vi "Main.vi"(11 "Module Admin":refnum<class "Delacor_lib_QMH_Module Admin.lvclass">) -> ()   [LabVIEW 2024, in "GUI.lvlib"]
doc: "This template is based off of the Queued Message Handler design pattern and the Queued Message Handler project template that ships with LabVIEW.\n\nThe main difference is that the queue is private to this module and communication between modules is performed via Broadcast and Request events.\n\nRequest events are wrapped in public API methods and are handled in the Event Handling Loop (EHL) of this VI. Any module can register for Broadcast events sent by this module. The EHL generates messages based on user interface actions.\n\nThe Message Handling Loop (MHL) processes messages generated by the EHL, or by other messages. The messages are string values, so new messages can be added easily to the Message Cases case structure in the MHL. Each message cluster can also provide an optional value for Message Data, which is a variant that can be converted to whatever message-specific data is required.\n_____\nBased on DQMH Project Template 7.0.1.1316."
uses:
  GUI.lvlib
  <vilib>/Delacor/Delacor QMH/Libraries/Module Admin_class/Delacor_lib_QMH_Module Admin.lvclass
  Module Data--cluster.ctl
  <vilib>/Delacor/Delacor QMH/Libraries/Message Queue_class/Delacor_lib_QMH_Message Queue.lvclass/Delacor_lib_QMH_Message Queue.ctl
  Stop Argument--cluster.ctl
  <vilib>/Delacor/Delacor QMH/Libraries/Module Admin_class/Delacor_lib_QMH_Module Admin.lvclass/Delacor_lib_QMH_Module Admin.ctl
  <vilib>/Utility/miscctls.llb/LVPointTypeDef.ctl
  <vilib>/Delacor/Delacor QMH/Libraries/Message Queue_class/Delacor_lib_QMH_Enqueue Message (Single).vi
  <vilib>/Delacor/Delacor QMH/Libraries/Module Admin_class/Delacor_lib_QMH_Get External Launch.vi
  <vilib>/Delacor/Delacor QMH/Libraries/Message Queue_class/Delacor_lib_QMH_Message Queue.lvclass
  <vilib>/addons/_JKI.lib/REST Client/classes/REST Client/REST Client.lvclass
  <vilib>/NI/Advanced HTTP Client/Header--Combo Box.ctl
  <vilib>/NI/Advanced HTTP Client/Session.lvclass
  <vilib>/addons/_JKI.lib/REST Client/classes/REST Client/HTTP Header.ctl
panel:
  in  "Current Status":bool
  out "error out":errorcluster
  out "Status":string
  in  "Simulate MHL Error":bool
  in  "Simulate EHL Error":bool
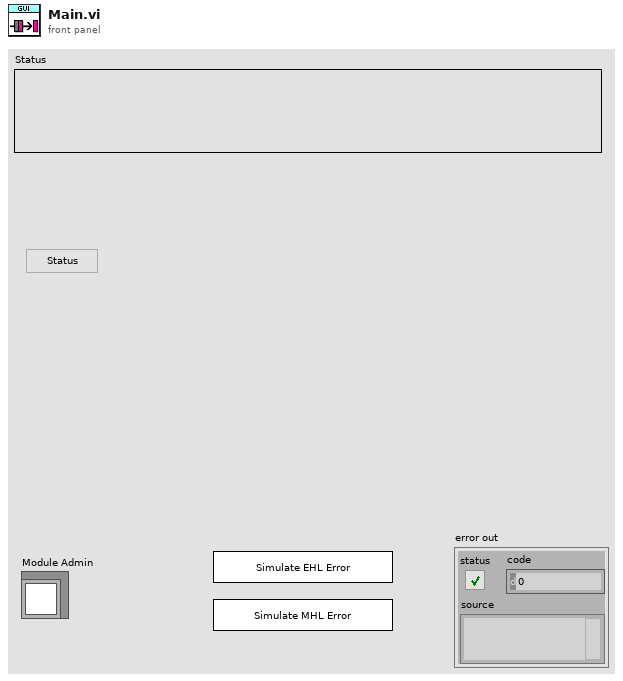
[diagram p1: front panel]
types:
  T1 = typedef "GUI.lvlib/Request Events--cluster.ctl" = cluster{"Stop Module":refnum<user-event>, "Show Panel":refnum<user-event>, "Hide Panel":refnum<user-event>, "Get Module Execution Status":refnum<user-event>, "Show Diagram":refnum<user-event>}
  T2 = typedef "GUI.lvlib/Module Data--cluster.ctl" = cluster{"Status":string, "Token":string, "Root Path":string, "REST Client":refnum<class "REST Client.lvclass">}
  T3 = enum32{"invalid lock state", "Not Locked", "Locked (No Password)", "Password-protected"}
  T4 = typedef "GUI.lvlib/Stop Argument--cluster.ctl" = cluster{"Origin":string, "Exit via Stop Module Req?":bool, "Wait for Module to stop?":bool}
  T5 = typedef "LVPointTypeDef.ctl" = cluster{"Horizontal":i16, "Vertical":i16}
  T6 = enum32{"Invalid", "Standard", "Closed", "Hidden", "Minimized", "Maximized"}
  T7 = typedef "lib_NI_Advanced HTTP Client.lvlib/Session.lvclass/Header--Combo Box.ctl" = string
  T8 = typedef "REST Client.lvlib/REST Client.lvclass/HTTP Header.ctl" = cluster{"header":T7, "value":string}
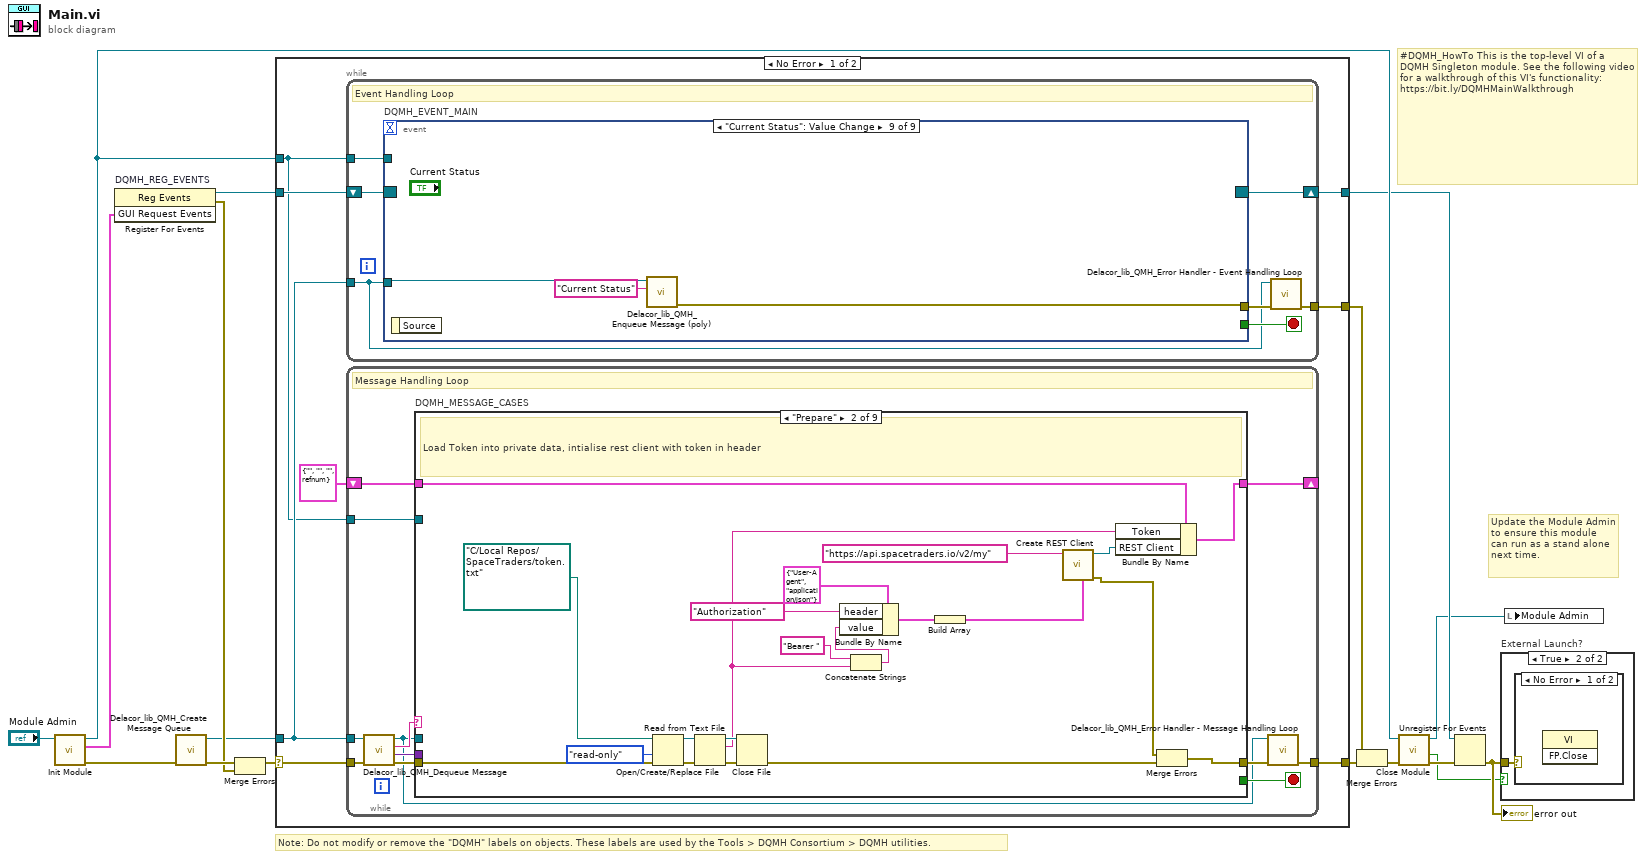
[diagram p0: block diagram]
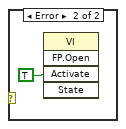
[diagram p3: hidden frame]
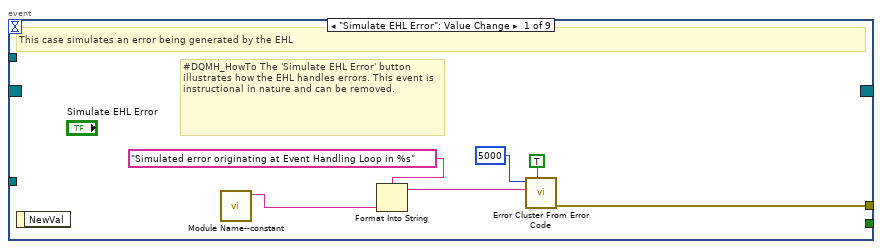
[diagram p4: hidden frame]
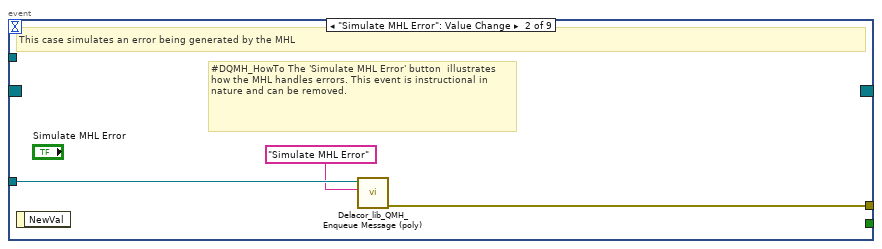
[diagram p5: hidden frame]
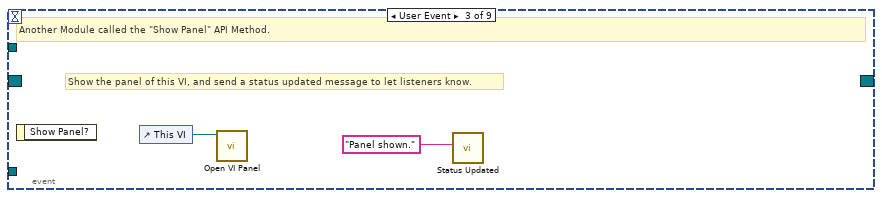
[diagram p6: hidden frame]
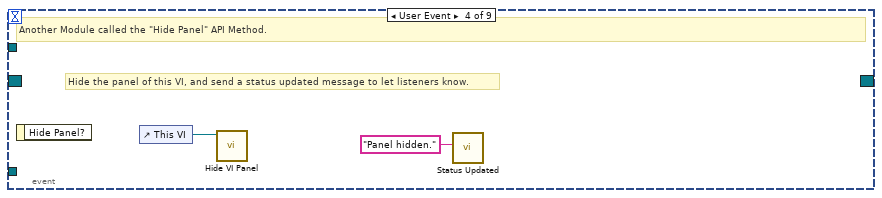
[diagram p7: hidden frame]
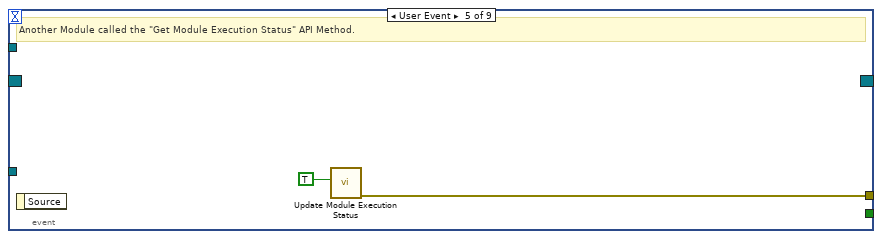
[diagram p8: hidden frame]
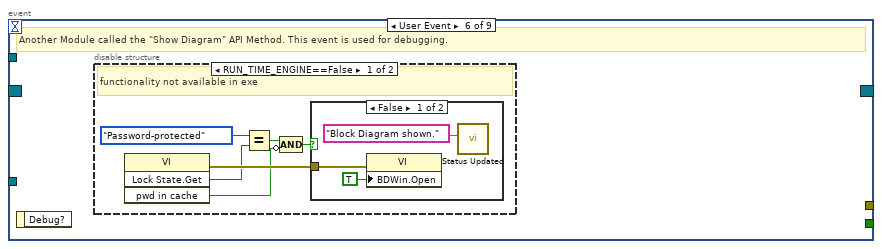
[diagram p9: hidden frame]
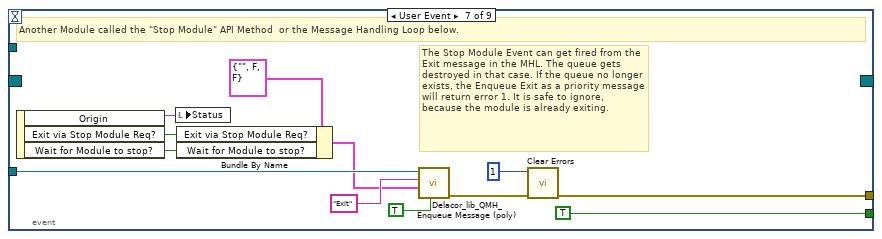
[diagram p12: hidden frame]
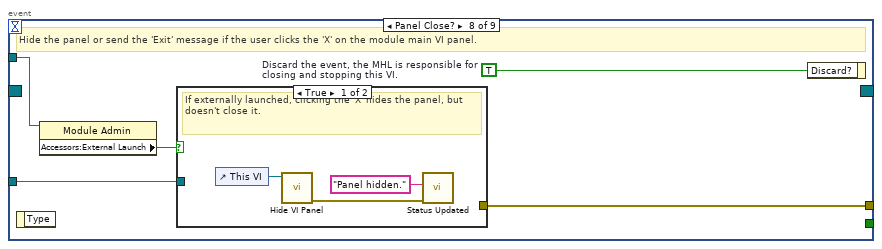
[diagram p13: hidden frame]
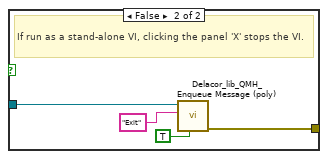
[diagram p14: hidden frame]
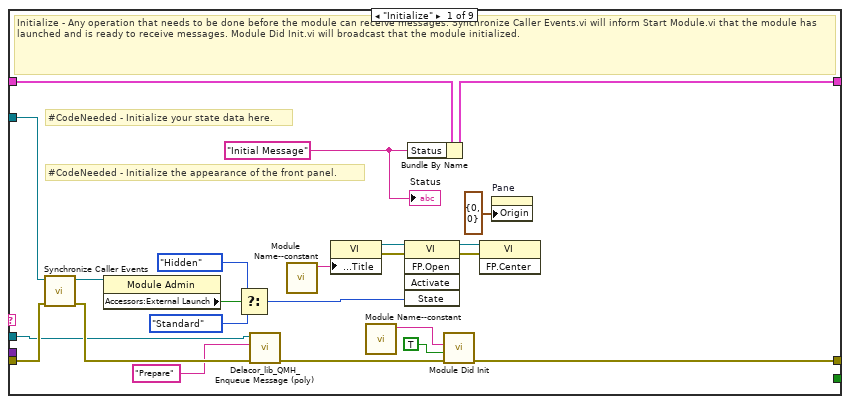
[diagram p15: hidden frame]
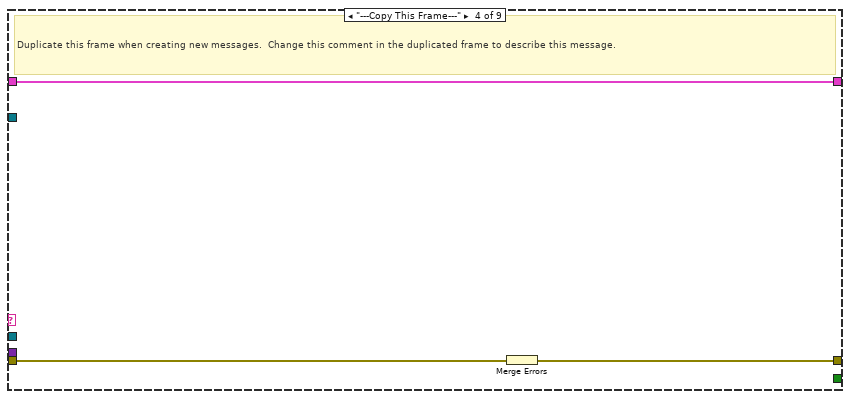
[diagram p17: hidden frame]
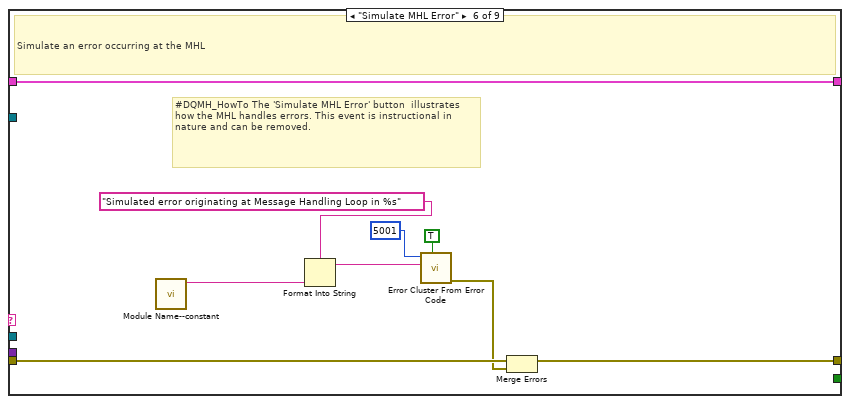
[diagram p19: hidden frame]
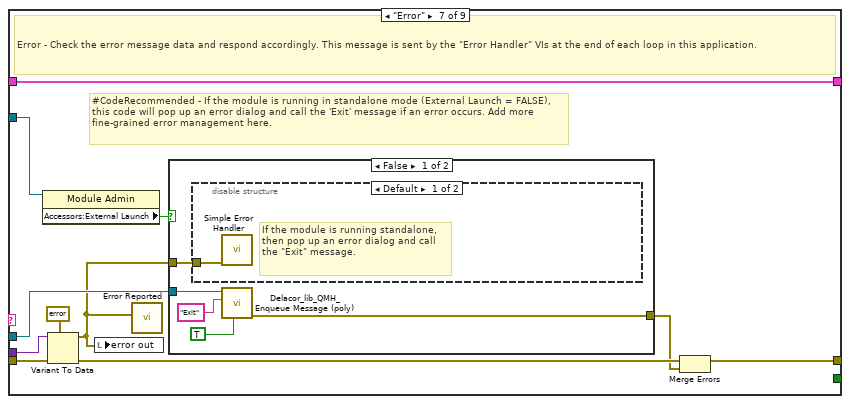
[diagram p20: hidden frame]
diagram:
  # "#DQMH_HowTo This is the top-level VI of a DQMH Singleton module. See the following video for a walkthrough of this VI's functionality: https://bit.ly/DQMHMainWalkthrough"
  # "Note: Do not modify or remove the \"DQMH\" labels on objects. These labels are used by the Tools > DQMH Consortium > DQMH utilities."
  # "Update the Module Admin to ensure this module can run as a stand alone next time."
  n1 = call "Init Module.vi"("Singleton Module Admin in"="Module Admin") -> ("error out"=w16:errorcluster, "GUI Request Events"=w5:T1, "Singleton Module Admin out"=w8:refnum<class "Delacor_lib_QMH_Module Admin.lvclass">)  [unwired: 8 in]
  n2 = register-events "DQMH_REG_EVENTS"(w5) -> (reference out=w6:refnum<event-registration>, error out=w9:errorcluster)  [unwired: 2 in]
  n3 = call <vilib>:"Delacor_lib_QMH_Create Message Queue.vi"("error in"=w16) -> ("error out"=w11:errorcluster, "Message Queue"=w4:refnum<class "Delacor_lib_QMH_Message Queue.lvclass">)  [unwired: 9 in]
  n4 = Merge Errors(w11, w9) -> (w10:errorcluster)
  n5 = case shown="No Error" w10 {
    selector: w10 -> [w23 w206]
    tunnel: [w25 w205] -> w17
    tunnel: [w22 w204] -> w7
    tunnel: w6 -> [w20 w204]
    tunnel: w4 -> [w19 w199]
    tunnel: [w24 _] -> w14
    tunnel: w8 -> [w18 w200]
    frame No Error {
      n6 = while {
        tunnel: w19 -> [w26]
        shift-right: [w29] -> w22
        shift-left: w20 -> [w30]
        tunnel: [w31] -> w24
        tunnel: w18 -> [w27]
        stop <- w28 stop-if-true
        # "Event Handling Loop"
        n7 = event "DQMH_EVENT_MAIN" shown="[8] \"Current Status\": Value Change" {
          selector: w30 -> [_ _ _ _ _ _ _ _ _]
          dyn-events: [_ _ _ _ _ _ _ _ _] -> w29
          timeout: _ -> [_ _ _ _ _ _ _ _ _]
          tunnel: [_ _ _ _ _ _ TRUE ("Discard?") _ _] -> w28
          tunnel: w26 -> [_ w40 _ _ _ _ w64 w71 w83]
          tunnel: [w38 w41 _ _ w47 _ w67 w73 w82] -> w32
          tunnel: w27 -> [_ _ _ _ _ _ _ w70 _]
          event "Simulate EHL Error": Value Change {
            # "#DQMH_HowTo The 'Simulate EHL Error' button  illustrates how the EHL handles errors. This event is instructional in nature and can be removed."
            # "This case simulates an error being generated by the EHL"
            n8 = event-data() -> ()  [unwired: 1 in, 1 out]
            n9 = call "Module Name--constant.vi"() -> ("Module Name"=w35:string)  [unwired: 11 in]
            n10 = Format Into String(format string="Simulated error originating at Event Handling Loop in %s", w35) -> (resulting string=w36:string)  [unwired: 2 in, 1 out]
            n11 = call <vilib>:"Error Cluster From Error Code.vi"("show call chain? (False)"=TRUE, "error message (\"\")"=w36, "error code (0)"=5000) -> ("error out"=w38:errorcluster)  [unwired: 6 in]
          }
          event "Simulate MHL Error": Value Change {
            # "#DQMH_HowTo The 'Simulate MHL Error' button  illustrates how the MHL handles errors. This event is instructional in nature and can be removed."
            # "This case simulates an error being generated by the MHL"
            n12 = event-data() -> ()  [unwired: 1 in, 1 out]
            n13 = call-poly <vilib>:"Delacor_lib_QMH_Enqueue Message (poly).vi"("Message"="Simulate MHL Error", "Message Queue in"=w40) -> ("error out"=w41:errorcluster)  [unwired: 8 in, 1 out]
          }
          event User Event {
            # "Show the panel of this VI, and send a status updated message to let listeners know."
            # "Another Module called the \"Show Panel\" API Method."
            n14 = event-data() -> ()  [unwired: 1 in, 1 out]
            n15 = control-ref of="This VI"() -> (w43:refnum<vi>)
            n16 = call "Open VI Panel.vi"("VI"=w43) -> ()  [unwired: 10 in, 1 out]
            n17 = call "Status Updated.vi"("Status"="Panel shown." ("format string")) -> ()  [unwired: 10 in, 1 out]
          }
          event User Event {
            # "Hide the panel of this VI, and send a status updated message to let listeners know."
            # "Another Module called the \"Hide Panel\" API Method."
            n18 = event-data() -> ()  [unwired: 1 in, 1 out]
            n19 = control-ref of="This VI"() -> (w45:refnum<vi>)
            n20 = call "Hide VI Panel.vi"("VI"=w45) -> ()  [unwired: 10 in, 1 out]
            n21 = call "Status Updated.vi"("Status"="Panel hidden." ("format string")) -> ()  [unwired: 10 in, 1 out]
          }
          event User Event {
            # "Another Module called the \"Get Module Execution Status\" API Method."
            n22 = event-data() -> ()  [unwired: 1 in, 1 out]
            n23 = call "Update Module Execution Status.vi"("Running?"=TRUE) -> ("error out"=w47:errorcluster)  [unwired: 10 in]
          }
          event User Event {
            # "Another Module called the \"Show Diagram\" API Method. This event is used for debugging."
            n24 = event-data() -> ()  [unwired: 1 in, 1 out]
            n25 = disable-structure shown="RUN_TIME_ENGINE==False" {
              frame condition #0 (active) {
                # "functionality not available in exe"
                n26 = invoke on="Invoke Node" class="VI" method="Lock State.Get"() -> (error out=w53:errorcluster, "Get Lock State"=w52:T3, "pwd in cache"=w49:bool)  [unwired: 4 in, 1 out]
                n27 = Equal?(x=T3."Password-protected", y=w52) -> (x = y?=w50:bool)
                n28 = Compound Arithmetic op=AND(w50, invert w49) -> (w48:bool)
                n29 = case shown="False" w48 {
                  tunnel: w53 -> [w56 _]
                  frame False {
                    n30 = property on="Property Node" class="VI"(error in=w56, "BDWin.Open"=TRUE ("Block Diagram Window:Open")) -> ()  [unwired: 1 in, 2 out]
                    n31 = call "Status Updated.vi"("Status"="Block Diagram shown." ("format string")) -> ()  [unwired: 10 in, 1 out]
                  }
                  frame True {
                    # "Password-protected VI, and the password is not in the cache. Do not show the diagram."
                  }
                }
              }
              frame condition #1 {
              }
            }
          }
          event User Event {
            # "The Stop Module Event can get fired from the Exit message in the MHL. The queue gets destroyed in that case. If the queue no longer exists, the Enqueue Exit as a priority message will return error 1. It is safe to ignore, because the module is already exiting."
            # "Another Module called the \"Stop Module\" API Method  or the Message Handling Loop below."
            n32 = event-data() -> ("Origin"=w63:string, "Exit via Stop Module Req?"=w59:bool, "Wait for Module to stop?"=w58:bool)  [unwired: 1 in]
            n33 = local write "Status"(w63) -> ()
            n34 = Bundle By Name(cluster=T4 {"Origin"="", "Exit via Stop Module Req?"=FALSE, "Wait for Module to stop?"=FALSE} ("Stop Argument"), "Exit via Stop Module Req?"=w59, "Wait for Module to stop?"=w58) -> (w57:T4)
            n35 = call-poly <vilib>:"Delacor_lib_QMH_Enqueue Message (poly).vi"("Priority Message? (F)"=TRUE, "Message Data"=w57, "Message"="Exit", "Message Queue in"=w64) -> ("error out"=w68:errorcluster)  [unwired: 6 in, 1 out]
            n36 = call <vilib>:"Clear Errors.vi"("error in (no error)"=w68, "specific error code to clear (0: all)"=1) -> ("error out"=w67:errorcluster)  [unwired: 4 in, 1 out]
          }
          event Panel Close? {
            w72 = TRUE  # Discard the event, the MHL is responsible for closing and stopping this VI.
            # "Hide the panel or send the 'Exit' message if the user clicks the 'X' on the module main VI panel."
            n37 = event-data() -> ()  [unwired: 1 in, 1 out]
            n38 = property on="Property Node" class="Module Admin"(reference=w70) -> ("Accessors:External Launch"=w69:bool)  [unwired: 1 in, 2 out]
            n39 = case shown="True" w69 {
              tunnel: w71 -> [_ w79]
              tunnel: [_ w80] -> w73
              frame True {
                # "If externally launched, clicking the 'X' hides the panel, but doesn't close it."
                n40 = control-ref of="This VI"() -> (w76:refnum<vi>)
                n41 = call "Hide VI Panel.vi"("VI"=w76) -> ("error out"=w74:errorcluster)  [unwired: 10 in]
                n42 = call "Status Updated.vi"("error in"=w74, "Status"="Panel hidden." ("format string")) -> ()  [unwired: 9 in, 1 out]
              }
              frame False {
                # "If run as a stand-alone VI, clicking the panel 'X' stops the VI."
                n43 = call-poly <vilib>:"Delacor_lib_QMH_Enqueue Message (poly).vi"("Priority Message? (F)"=TRUE, "Message"="Exit", "Message Queue in"=w79) -> ("error out"=w80:errorcluster)  [unwired: 7 in, 1 out]
              }
            }
            n44 = event-data ("Event Filter Node")("Discard?"=w72) -> ()  [unwired: 1 in, 1 out]
          }
          event "Current Status": Value Change {
            n45 = event-data() -> ()  [unwired: 1 in, 1 out]
            n46 = call-poly <vilib>:"Delacor_lib_QMH_Enqueue Message (poly).vi"("Message"="Current Status", "Message Queue in"=w83) -> ("error out"=w82:errorcluster)  [unwired: 8 in, 1 out]
          }
        }
        n47 = call-dynamic "Delacor_lib_QMH_Error Handler - Event Handling Loop.vi"("error in"=w32, "Message Queue in"=w26) -> ("dup error in"=w31:errorcluster)  [unwired: 8 in, 1 out]
      }
      n48 = while {
        tunnel: w19 -> [w84]
        shift-right: [w92] -> _
        shift-left: T2 {"Status"="", "Token"="", "Root Path"="", "REST Client"=refnum} ("Data Cluster") -> [w93]
        tunnel: w23 -> [w95]
        tunnel: [w87] -> w25
        tunnel: w18 -> [w88]
        stop <- w91 stop-if-true
        # "Message Handling Loop"
        n49 = call-dynamic "Delacor_lib_QMH_Dequeue Message.vi"("error in"=w95, "Message Queue in"=w84) -> ("error out"=w94:errorcluster, "Message Data"=w89:variant, "Message"=w90:string, "Message Queue out"=w85:refnum<class "Delacor_lib_QMH_Message Queue.lvclass">)  [unwired: 6 in]
        n50 = case "DQMH_MESSAGE_CASES" shown="\"Prepare\"" w90 {
          selector: w90 -> [_ _ _ _ _ _ _ _ w194]
          tunnel: w85 -> [w97 _ _ _ _ _ w159 w182 _]
          tunnel: w94 -> [w116 w131 w141 w144 w146 w155 w166 w188 w197]
          tunnel: [w114 w127 w141 w143 w146 w154 w162 w183 w198] -> w86
          tunnel: w93 -> [w105 w134 w140 w142 w145 w152 w161 w174 w195]
          tunnel: [w104 w133 w140 w142 w145 w152 w161 w174 w195] -> w92
          tunnel: [_ _ _ _ _ _ _ w181 _] -> w91
          tunnel: w89 -> [_ _ _ _ _ _ w160 w180 _]
          tunnel: w88 -> [w106 _ _ _ _ _ w158 w175 _]
          frame "Initialize" {
            w100 = "Initial Message" ("Initial Message")
            # "#CodeNeeded - Initialize the appearance of the front panel."
            # "#CodeNeeded - Initialize your state data here."
            # "Initialize - Any operation that needs to be done before the module can receive messages. Synchronize Caller Events.vi will inform Start Module.vi that the module has launched and is ready to receive messages. Module Did Init.vi will broadcast that the module initialized."
            n51 = call "Synchronize Caller Events.vi"("error in"=w116, "Singleton Module Admin in"=w106) -> ("error out"=w115:errorcluster, "Singleton Module Admin out"=w101:refnum<class "Delacor_lib_QMH_Module Admin.lvclass">)  [unwired: 8 in]
            n52 = property on="Property Node" class="Module Admin"(reference=w101) -> ("Accessors:External Launch"=w110:bool)  [unwired: 1 in, 2 out]
            n53 = Select(t=T6."Hidden" ("State"), s=w110, f=T6."Standard" ("State")) -> (s? t:f=w107:T6)
            n54 = call-poly <vilib>:"Delacor_lib_QMH_Enqueue Message (poly).vi"("error in"=w115, "Message"="Prepare", "Message Queue in"=w97) -> ("error out"=w98:errorcluster)  [unwired: 7 in, 1 out]
            n55 = call "Module Name--constant.vi"() -> ("Module Name"=w113:string)  [unwired: 11 in]
            n56 = property on="Property Node" class="VI"("Front Panel.Title"=w113) -> (reference out=w112:refnum<vi>, error out=w118:errorcluster)  [unwired: 2 in]
            n57 = call "Module Name--constant.vi"() -> ("Module Name"=w102:string)  [unwired: 11 in]
            n58 = invoke on="Invoke Node" class="VI" method="FP.Open"(reference=w112, error in=w118, "State"=w107) -> (reference out=w111:refnum<vi>, error out=w117:errorcluster)  [unwired: 2 in, 3 out]
            n59 = Bundle By Name(cluster=w105, "Status"=w100) -> (w104:T2)
            n60 = call "Module Did Init.vi"("error in"=w98, "Initialized?"=TRUE, "Origin"=w102) -> ("error out"=w114:errorcluster)  [unwired: 8 in]
            n61 = invoke on="Invoke Node" class="VI" method="FP.Center"(reference=w111, error in=w117) -> ()  [unwired: 1 in, 3 out]
            n62 = property on="Pane" class="Pane"("Origin"=T5 {"Horizontal"=0, "Vertical"=0}) -> ()  [unwired: 2 in, 2 out]
            "Status" <- w100
          }
          frame "Prepare" {
            # "Load Token into private data, intialise rest client with token in header"
            n63 = Open/Create/Replace File(file path (use dialog)=path "C:/Local Repos/SpaceTraders/token.txt", error in=w131, access (0:read/write)=enum16{"read/write", "read-only", "write-only"}."read-only") -> (refnum out=w139:refnum<file>, error out=w138:errorcluster)  [unwired: 3 in, 1 out]
            n64 = Read from Text File(file (use dialog)=w139, error in=w138) -> (refnum out=w137:refnum<file>, text=w119:string, error out=w136:errorcluster)  [unwired: 2 in, 1 out]
            n65 = Close File(refnum=w137, error in=w136) -> (error out=w132:errorcluster)  [unwired: 1 out]
            n66 = Concatenate Strings("Bearer ", w119) -> (w121:string)
            n67 = Bundle By Name(cluster=T8 {"header"="User-Agent", "value"="application/json"} ("Header"), "header"=T7 "Authorization", "value"=w121) -> (w123:T8)
            n68 = Build Array(w123) -> (w122:T8[])
            n69 = call <vilib>:"Create REST Client.vi"("Default Headers ([JSON])"=w122, "Base URL"="https://api.spacetraders.io/v2/my" ("Root Path")) -> ("error out"=w126:errorcluster, "REST Client out"=w128:refnum<class "REST Client.lvclass">)  [unwired: 8 in]
            n70 = Bundle By Name(cluster=w134, "Token"=w119, "REST Client"=w128) -> (w133:T2)
            n71 = Merge Errors(w126, w132) -> (w127:errorcluster)
          }
          frame "---Module Specific---" {
            # "Separator -- The following cases handle messages specific to this Module."
          }
          frame "---Copy This Frame---" {
            # "Duplicate this frame when creating new messages.  Change this comment in the duplicated frame to describe this message."
            n72 = Merge Errors(w144) -> (w143:errorcluster)
          }
          frame "---Exit and Error Handling---" {
            # "Separator - The following cases handle errors and exit messages."
          }
          frame "Simulate MHL Error" {
            # "#DQMH_HowTo The 'Simulate MHL Error' button  illustrates how the MHL handles errors. This event is instructional in nature and can be removed."
            # "Simulate an error occurring at the MHL"
            n73 = call "Module Name--constant.vi"() -> ("Module Name"=w148:string)  [unwired: 11 in]
            n74 = Format Into String(format string="Simulated error originating at Message Handling Loop in %s", w148) -> (resulting string=w149:string)  [unwired: 2 in, 1 out]
            n75 = call <vilib>:"Error Cluster From Error Code.vi"("show call chain? (False)"=TRUE, "error message (\"\")"=w149, "error code (0)"=5001) -> ("error out"=w153:errorcluster)  [unwired: 6 in]
            n76 = Merge Errors(w155, w153) -> (w154:errorcluster)
          }
          frame "Error" {
            # "#CodeRecommended - If the module is running in standalone mode (External Launch = FALSE), this code will pop up an error dialog and call the 'Exit' message if an error occurs. Add more fine-grained error management here."
            # "Error - Check the error message data and respond accordingly. This message is sent by the \"Error Handler\" VIs at the end of each loop in this application."
            n77 = property on="Property Node" class="Module Admin"(reference=w158) -> ("Accessors:External Launch"=w157:bool)  [unwired: 1 in, 2 out]
            n78 = Variant To Data(error in=w166, type=errorcluster {"status"=FALSE, "code"=0, "source"=""} ("error constant"), Variant=w160) -> (data=w156:errorcluster, error out=w164:errorcluster)
            n79 = local write "error out"(w156) -> ()
            n80 = call "Error Reported.vi"("Error"=w156) -> ()  [unwired: 10 in, 1 out]
            n81 = case shown="False" w157 {
              tunnel: [w171 _] -> w163
              tunnel: w159 -> [w169 _]
              tunnel: w156 -> [w170 _]
              frame False {
                n82 = disable-structure shown="Default" {
                  disable-tunnel: w170 -> [w172 _]
                  frame condition #0 (active) {
                    # "If the module is running standalone, then pop up an error dialog and call the \"Exit\" message."
                    n83 = call <vilib>:"Simple Error Handler.vi"("error in (no error)"=w172) -> ()  [unwired: 4 in, 5 out]
                  }
                  frame condition #1 {
                    # "To prevent the Simple Error Handler VI from being loaded (e.g. when deploying to a Real-Time target), add the Conditional Disable Symbol \"DQMH_Disable_SEH\" to your project and set it to TRUE."
                  }
                }
                n84 = call-poly <vilib>:"Delacor_lib_QMH_Enqueue Message (poly).vi"("Priority Message? (F)"=TRUE, "Message"="Exit", "Message Queue in"=w169) -> ("error out"=w171:errorcluster)  [unwired: 7 in, 1 out]
              }
              frame True {
                # "If the module was launched externally, calling the Error Reported broadcast VI is the only action performed by the \"Error\" message. The module's caller can then process the error appropriately."
              }
            }
            n85 = Merge Errors(w164, w163) -> (w162:errorcluster)
          }
          frame "Exit" {
            w179 = 91  # 91: not all Exit messages will have an argument
            w181 = TRUE  # Stop the VI
            # "Release the message queue reference"
            # "#CodeNeeded - Add any required cleanup code here."
            # "Exit - Exit the application."
            n86 = Variant To Data(error in=w188, type=T4 {"Origin"="", "Exit via Stop Module Req?"=FALSE, "Wait for Module to stop?"=FALSE} ("Stop Argument"), Variant=w180) -> (data=w177:T4, error out=w185:errorcluster)
            n87 = call <vilib>:"Clear Errors.vi"("error in (no error)"=w185, "specific error code to clear (0: all)"=w179) -> ("error out"=w187:errorcluster)  [unwired: 4 in, 1 out]
            n88 = control-ref of="This VI"() -> (w176:refnum<vi>)
            n89 = call-dynamic "Delacor_lib_QMH_Release Message Queue.vi"("error in"=w187, "Message Queue"=w182) -> ("error out"=w186:errorcluster)  [unwired: 9 in]
            n90 = call "Handle Exit.vi"("Stop Argument"=w177, "Admin in"=w175, "VI reference"=w176) -> ("error out"=w184:errorcluster)  [unwired: 7 in, 1 out]
            n91 = Merge Errors(w186, w184) -> (w183:errorcluster)
            n92 = Unbundle By Name(w174) -> ("REST Client"=w173:refnum<class "REST Client.lvclass">)
            n93 = call "Error Reported.vi"("Error"=w183) -> ()  [unwired: 10 in, 1 out]
            n94 = call-dynamic "Destroy REST Client.vi"("REST Client in"=w173) -> ()  [unwired: 10 in, 1 out]
          }
          frame Default {
            # "'Default' case only runs if there is a message that isn't defined in any of the other cases.  Output a programming error."
            n95 = call "Module Name--constant.vi"() -> ("Module Name"=w193:string)  [unwired: 11 in]
            n96 = Format Into String(format string="The invalid message string \"%s\" was received in the Message Handling Loop for module \"%s\".", w194, w193) -> (resulting string=w189:string)  [unwired: 2 in, 1 out]
            n97 = call <vilib>:"Error Cluster From Error Code.vi"("show call chain? (False)"=TRUE, "error message (\"\")"=w189, "error code (0)"=1) -> ("error out"=w196:errorcluster)  [unwired: 6 in]
            n98 = Merge Errors(w197, w196) -> (w198:errorcluster)
          }
        }
        n99 = call-dynamic "Delacor_lib_QMH_Error Handler - Message Handling Loop.vi"("error in"=w86, "Message Queue in"=w85) -> ("dup error in"=w87:errorcluster)  [unwired: 8 in, 1 out]
      }
    }
    frame Error {
      # "Synchronize Caller Events.vi will inform Start Module.vi that the module has launched and will let the code calling Start Module.vi register for broadcasts and would permit the caller receive the broadcast that an error occurred at launch time."
      n100 = call-dynamic "Delacor_lib_QMH_Release Message Queue.vi"("error in"=w206, "Message Queue"=w199) -> ("error out"=w205:errorcluster)  [unwired: 9 in]
      n101 = call "Synchronize Caller Events.vi"("Singleton Module Admin in"=w200) -> ("error out"=w207:errorcluster)  [unwired: 9 in, 1 out]
      n102 = call "Module Name--constant.vi"() -> ("Module Name"=w203:string)  [unwired: 11 in]
      n103 = Format Into String(format string="An error occurred during initialization. %s is no longer running.", w203) -> (resulting string=w201:string)  [unwired: 2 in, 1 out]
      n104 = Merge Errors(w205, w207) -> (w208:errorcluster)
      n105 = call "Error Reported.vi"("Additional Information"=w201, "Error"=w208) -> ()  [unwired: 9 in, 1 out]
    }
  }
  n106 = Merge Errors(w14, w17) -> (w13:errorcluster)
  n107 = call "Close Module.vi"("error in"=w13, "Module Admin in"=w8) -> ("error out"=w15:errorcluster, "External Launch"=w1:bool, "Module Admin out"=w2:refnum<class "Delacor_lib_QMH_Module Admin.lvclass">)  [unwired: 7 in]
  n108 = Unregister For Events(event registration refnum=w7, error in=w15) -> (error out=w12:errorcluster)
  "error out" <- w12
  n109 = case "External Launch?" shown="True" w1 {
    tunnel: w12 -> [_ w209]
    frame False {
    }
    frame True {
      n110 = case shown="No Error" w209 {
        frame No Error {
          n111 = invoke on="Invoke Node" class="VI" method="FP.Close"() -> ()  [unwired: 3 in, 3 out]
        }
        frame Error {
          n112 = invoke on="Invoke Node" class="VI" method="FP.Open"("Activate"=TRUE ("Activate?")) -> ()  [unwired: 4 in, 5 out]
        }
      }
    }
  }
  n113 = local write "Module Admin"(w2) -> ()
